vi "All Keyed Array VIs.vi"() -> ()   [LabVIEW 2009, in "Tools_KeyedArray.lvlib"]
uses:
  Tools_KeyedArray.lvlib
panel:
  out "KA XML Children":string
  out "KA String":string
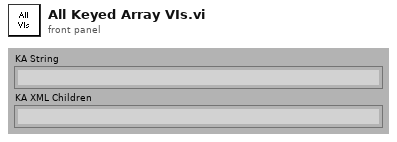
[diagram p1: front panel]
types:
  T1 = typedef "Tools_KeyedArray.lvlib/KeyedArray.ctl" = cluster{"keys":string[], "values":string[]}
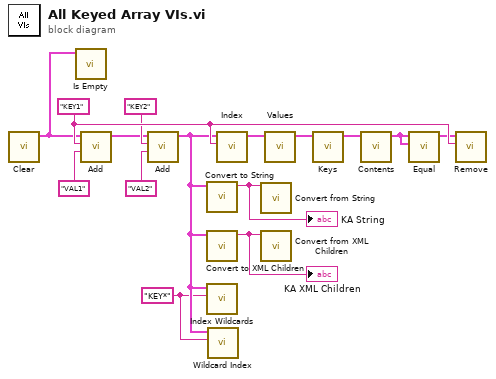
[diagram p0: block diagram]
diagram:
  w2 = "KEY*" ("key")
  w11 = "KEY1" ("key")
  n1 = call "Clear.vi"() -> ("array out"=w1:T1)  [unwired: 1 in, 6 out]
  n2 = call "Is Empty.vi"("array in"=w1) -> ()  [unwired: 7 out]
  n3 = call "Add.vi"("value"="VAL1" ("key"), "key"=w11, "array in"=w1) -> ("array out"=w4:T1)  [unwired: 1 in, 3 out]
  n4 = call "Add.vi"("value"="VAL2" ("key"), "key"="KEY2", "array in"=w4) -> ("array out"=w3:T1)  [unwired: 1 in, 3 out]
  n5 = call "Convert to String.vi"("keyed array"=w3) -> ("KA string"=w8:string)  [unwired: 10 out]
  "KA String" <- w8
  n6 = call "Convert to XML Children.vi"("keyed array"=w3) -> ("KA XML children"=w7:string)  [unwired: 10 out]
  "KA XML Children" <- w7
  n7 = call "Index Wildcards.vi"("key"=w2, "array in"=w3) -> ()  [unwired: 2 in, 4 out]
  n8 = call "Wildcard Index.vi"("wildcard key"=w2, "array in"=w3) -> ()  [unwired: 2 in, 4 out]
  n9 = call "Index.vi"("key"=w11, "array in"=w3) -> ("duplicate array"=w15:T1)  [unwired: 2 in, 3 out]
  n10 = call "Convert from String.vi"("KA string"=w8) -> ()  [unwired: 1 in, 10 out]
  n11 = call "Convert from XML Children.vi"("KA string"=w7) -> ()  [unwired: 1 in, 10 out]
  n12 = call "Values.vi"("array in"=w15) -> ("duplicate array"=w14:T1)  [unwired: 6 out]
  n13 = call "Keys.vi"("array in"=w14) -> ("duplicate array"=w13:T1)  [unwired: 6 out]
  n14 = call "Contents.vi"("array in"=w13) -> ("duplicate array"=w9:T1)  [unwired: 6 out]
  n15 = call "Equal.vi"("array B"=w9, "array A"=w9) -> ("duplicate array A"=w10:T1)  [unwired: 2 in, 3 out]
  n16 = call "Remove.vi"("key"=w11, "array in"=w10) -> ()  [unwired: 1 in, 5 out]
